vi "ConfigurationGetKeysRequest_Name.vi"() -> (1 "MessageName":string)   [LabVIEW 2017]
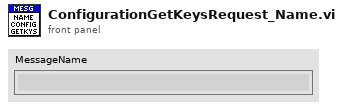
[diagram p1: front panel]
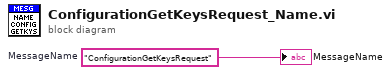
[diagram p0: block diagram]
diagram:
  w1 = "ConfigurationGetKeysRequest"  # MessageName
  "MessageName" <- w1
